vi "Test Missing Libraries.vi"(11 "Test Case In":refnum<class "Missing in Project.lvclass">) -> (0 "error out":errorcluster, 3 "Test Case Out":refnum<class "Missing in Project.lvclass">)   [LabVIEW 2021, in "Missing in Project.lvclass"]
doc: "Tests to make sure all libraries defined in the project are saved to disk."
uses:
  Missing in Project.lvclass
  <vilib>/Astemes/LUnit/Test Case.lvclass/Test Case.ctl
  <vilib>/Astemes/LUnit/Append Pass Result.vi
  <vilib>/Astemes/LUnit/Append Fail Result.vi
  <vilib>/Astemes/LUnit/Run In UI.vi
  <vilib>/Utility/error.llb/Clear Errors.vi
  Missing in Project.lvclass/Missing in Project.ctl
  <vilib>/Astemes/LUnit/Test Case.lvclass
  C:/Program Files/National Instruments/LabVIEW 2021/vi.lib/Astemes/LUnit/Test Case.lvclass
  C:/Program Files/National Instruments/LabVIEW 2021/vi.lib/Astemes/LUnit/LUnit Runnable.lvclass
  C:/Users/J63553/Projects/_LabVIEW Community/labview-icon-editor-unit-tests/Tooling/Unit tests/Missing in Project/Missing in Project.lvclass
panel:
  out "Missing items from LabVIEW project":path[](array[path])
  out "Pass":bool
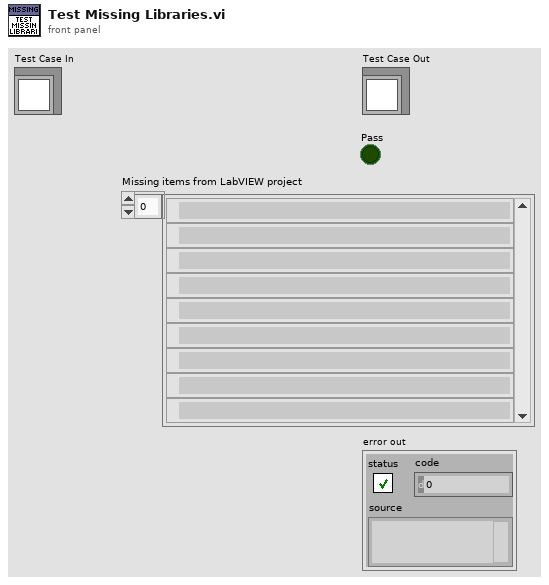
[diagram p1: front panel]
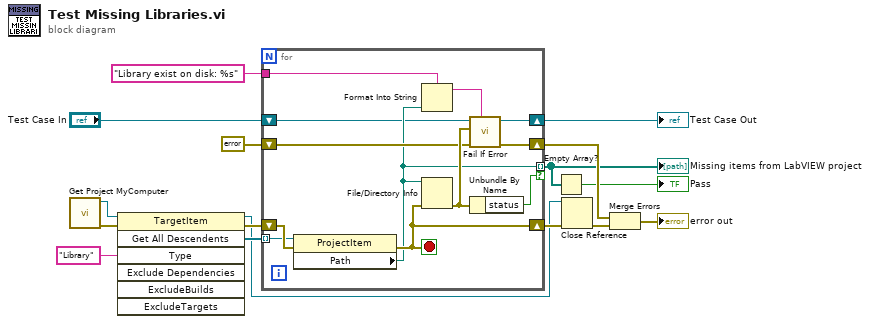
[diagram p0: block diagram]
diagram:
  n1 = call "Get Project MyComputer.vi"() -> ("error out"=w12:errorcluster, "My Computer"=w4:refnum<vi>)  [unwired: 10 in]
  n2 = invoke class="TargetItem" method="Get All Descendents"(reference=w4, error in=w12, "Type"="Library") -> (reference out=w7:refnum<vi>, error out=w16:errorcluster, "All Descendents"=w8:refnum<vi>[])  [unwired: 4 in, 4 out]
  n3 = for {
    tunnel: w8 -> [w23] mode=indexing
    shift-right: [w26] -> w15
    shift-left: w16 -> [w27]
    tunnel: [w22] -> w5 mode=indexing if=w19
    shift-right: [w24] -> w10
    shift-left: errorcluster {"status"=FALSE, "code"=0, "source"=""} ("error in (no error)") -> [w25]
    shift-right: [w21] -> w2
    shift-left: "Test Case In" -> [w20]
    tunnel: "Library exist on disk: %s" ("Label") -> [w18]
    stop <- w26 stop-if-true
    n4 = property class="ProjectItem"(reference=w23, error in=w27) -> (error out=w26:errorcluster, "Path"=w22:path)  [unwired: 1 out]
    n5 = Format Into String(format string=w18, w22) -> (resulting string=w17:string)  [unwired: 2 in, 1 out]
    n6 = File/Directory Info(path=w22, error in=w26) -> (error out=w28:errorcluster)  [unwired: 6 out]
    n7 = call <vilib>:"Fail If Error.vi"("Description"=w17, "error in (no error)"=w25, "Assert error"=w28, "LUnit Test Case In"=w20) -> ("error out"=w24:errorcluster, "LUnit Test Case Out"=w21:refnum<class "Missing in Project.lvclass">)  [unwired: 6 in]
    n8 = Unbundle By Name(w28) -> ("status"=w19:bool)
  }
  "Missing items from LabVIEW project" <- w5
  "Test Case Out" <- w2
  n9 = Empty Array?(array=w5) -> (empty?=→"Pass":bool)
  n10 = Close Reference(reference=w7, error in (no error)=w15) -> (error out=w14:errorcluster)
  n11 = Merge Errors(w10, w14) -> (→"error out":errorcluster)
